vi "FTW-FileSystem-OpenDirectoryOrParent.vi"(0 "Directory to Open":path, 11 "error in":errorcluster) -> (4 "Directory Actually Opened":path, 15 "error out":errorcluster)   [LabVIEW 2013]
panel:
  # "Inputs"
  # "Outputs"
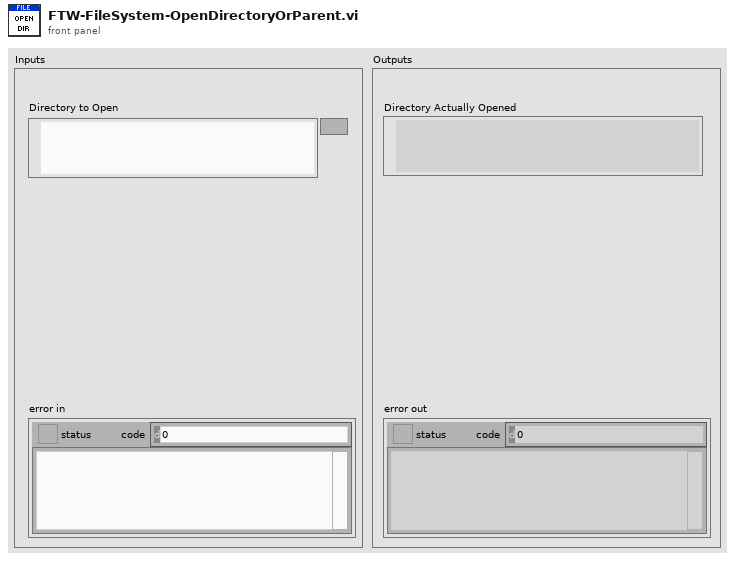
[diagram p1: front panel]
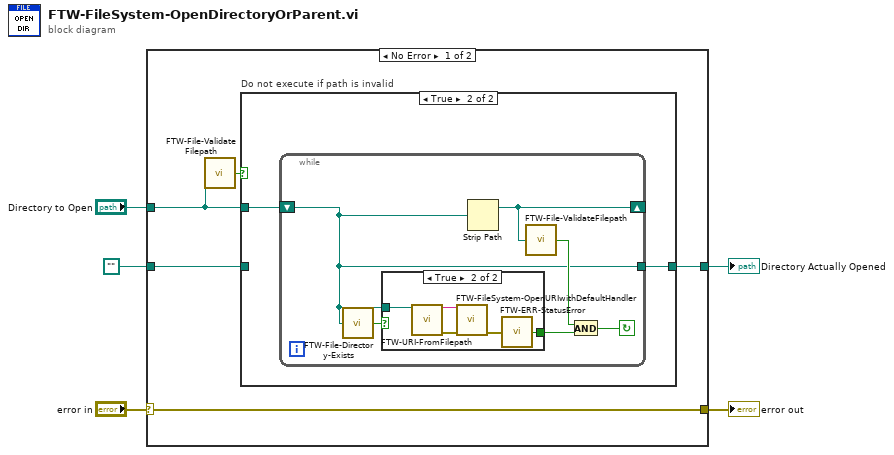
[diagram p0: block diagram]
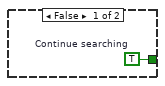
[diagram p3: hidden frame]
diagram:
  n1 = case shown="No Error" "error in" {
    selector: "error in" -> [w6 w27]
    tunnel: "Directory to Open" -> [w8 _]
    tunnel: [w10 w26] -> w4
    tunnel: [w6 w27] -> w2
    tunnel: path "" -> [w9 w26]
    frame No Error {
      n2 = call "FTW-File-ValidateFilepath.vi"("Filepath"=w8) -> ("Valid?"=w7:bool)
      n3 = case "Do not execute if path is invalid" shown="True" w7 {
        tunnel: w8 -> [_ w13]
        tunnel: [w11 w12] -> w10
        tunnel: w9 -> [w11 _]
        frame False {
        }
        frame True {
          n4 = while {
            shift-right: [w19] -> _
            shift-left: w13 -> [w15]
            tunnel: [w15] -> w12
            stop <- w17 continue-if-true
            n5 = call "FTW-File-Directory-Exists.vi"("Directory"=w15) -> ("Exists?"=w14:bool)
            n6 = case shown="True" w14 {
              tunnel: [w20 w22] -> w16
              tunnel: w15 -> [_ w21]
              frame False {
                w20 = TRUE  # Continue searching
              }
              frame True {
                n7 = call "FTW-URI-FromFilepath.vi"("Path"=w21) -> ("URI"=w25:string, "error out"=w24:errorcluster)  [unwired: 13 in]
                n8 = call "FTW-FileSystem-OpenURIwithDefaultHandler.vi"("URI to Open"=w25, "error in"=w24) -> ("error out"=w23:errorcluster)  [unwired: 12 in, 1 out]
                n9 = call "FTW-ERR-StatusError.vi"("error to check"=w23) -> ("Error?"=w22:bool)
              }
            }
            n10 = Strip Path(path=w15) -> (stripped path=w19:path)  [unwired: 1 out]
            n11 = call "FTW-File-ValidateFilepath.vi"("Filepath"=w19) -> ("Valid?"=w18:bool)
            n12 = And(x=w18, y=w16) -> (x .and. y?=w17:bool)
          }
        }
      }
    }
    frame Error {
    }
  }
  "error out" <- w2
  "Directory Actually Opened" <- w4
